vi "1473R Acquisition Template (Host).vi"() -> ()   [LabVIEW 2015]
uses:
  <vilib>/rvi/interface/nirviOpenFPGA/nirviOpenFPGA.xnode
  <vilib>/rvi/interface/nirviMethod/nirviMethod.xnode
  <vilib>/rvi/interface/nirviReadWriteControl/nirviReadWriteControl.xnode
  <vilib>/rvi/interface/nirviCloseFPGA/nirviCloseFPGA.xnode
  <vilib>/rvi/interface/Simulation/niFpgaSimulationCallBeginRW.vi
  <vilib>/rvi/errors/niLvFpgaAdjustHostInterfaceError.vi
  <vilib>/FPGAPlugInAG/Dynamic/niLvFpga_Run_Dynamic.vi
  <vilib>/FPGAPlugInAG/Dynamic/niLvFpga_Close_Dynamic.vi
  <vilib>/visionFPGA/NI_VDM_FPGA_Basics.lvlib
  <vilib>/visionFPGA/Basics/Configure Image Transfer from Target/IMAQ FPGA Configure Image Transfer from Target U8.vi
  <vilib>/FPGAPlugInAG/Dynamic/niLvFpga_Download_Dynamic.vi
  <vilib>/visionFPGA/Basics/Image Transfer from Target/IMAQ FPGA Image Transfer from Target U8.vi
  NiFpgaLv.dll
  <vilib>/Utility/error.llb/Error Cluster From Error Code.vi
  FPGA Bitfiles/ImageProcessingw_FPGATarget1_ImageProcessingw_ENrq3A+Q5NY.lvbitx
  Image Processing with Vision Assistant on 1473R (FPGA).vi
  <vilib>/FPGAPlugInAG/PCIe-1473R/niLvFpga_Open_PCIe-1473R.vi
  <vilib>/rvi/interface/common/dynamic/niFpgaDynamicAddResources.vi
  <vilib>/userdefined/Silver/nirio_resource_slv.ctl
panel:
  in  "Image Size":cluster{"Height":u32, "Width":u32}
  out "Acq In Progress":bool
  in  "Line Scan":bool
  in  "Frames To Acquire":u32=1 caption="Frames To Acquire\n(0 = infinite)"
  in  "Cancel":bool
  out "Acq'd Frame Width":u32
  in  "Stopped":bool
  in  "RIO Device":T1="RIO0"
  out "Acquisition Overflow":bool
  in  "Start Serial Server":bool=TRUE
  out "Frames Acq'd":u32
  out "Acq'd Frame Height":u32
  out "Image":T2(plugin-control)
  in  "Acquire":bool
  in  "Stop":bool
  out "Initialized":bool
  # "Overview: Demonstrates how to acquire an image from a Camera Link camera using the 1473R, process the image on the FPGA using the Vision Assistant Express VI, and transfer the processed image to the host.  Additionally, the example demonstrates the serial server, which allows third-party camera configuration utilities to communicate with the camera using the Camera Link serial interface while this VI is running.\nRequirements:\n- LabVIEW FPGA\n- Vision Acquisition Software\n- Vision Development Module\nInstructions:\n1. Select the RIO Device corresponding to the 1473R.\n2. Set the image size controls to the expected size of the image from the camera.\n3. Run the VI."
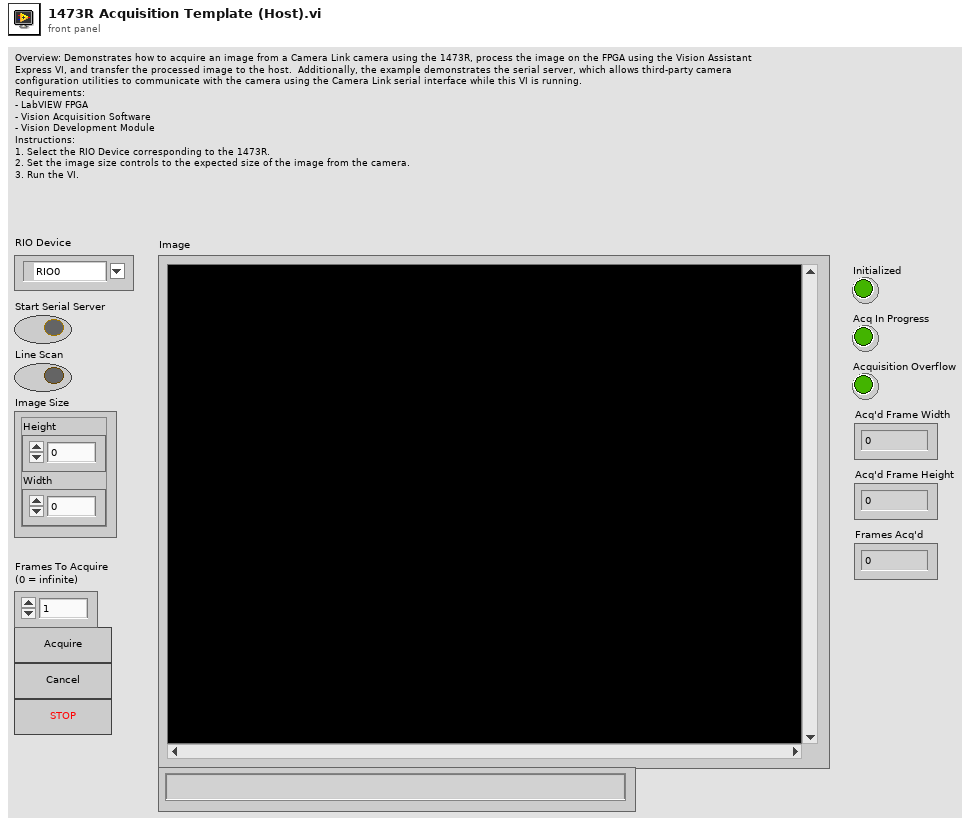
[diagram p1: front panel]
types:
  T1 = typedef "nirio_resource_slv.ctl" = tag
  T2 = typedef "IMAQ Image.ctl" = refnum<image>
  T3 = enum8{"Standard", "Basler 10-tap", "Vosskühler 10-tap"}
  T4 = typedef "Image Type" = u32
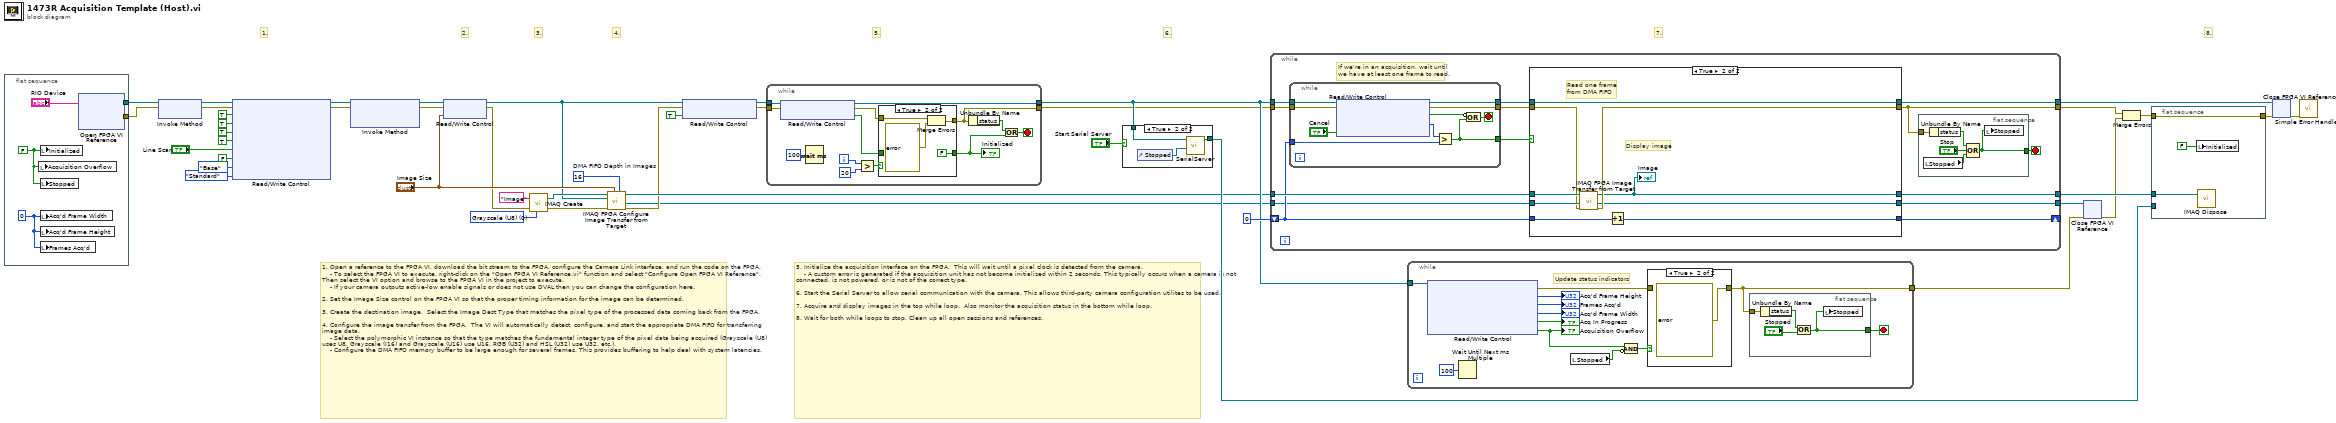
[diagram p0: block diagram]
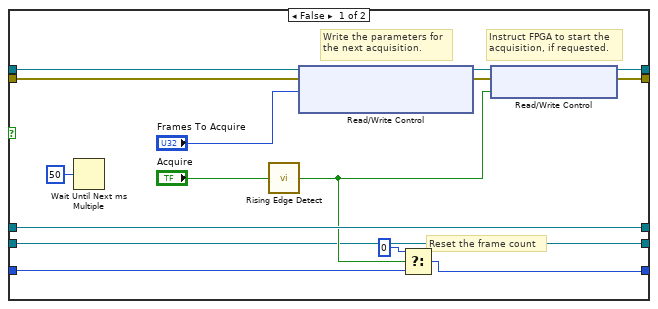
[diagram p4: hidden frame]
diagram:
  w12 = u32 16  # DMA FIFO Depth in Images
  w40 = T4 0 items=["Grayscale (U8)", "Grayscale (I16)", "Grayscale (SGL)", "Complex (CSG)", "RGB (U32)", "HSL (U32)", "RGB (U64)", "Grayscale (U16)"] ("Image Type")
  # "8."
  # "7."
  # "6."
  # "5."
  # "4."
  # "3."
  # "2."
  # "1."
  # "5. Initialize the acquisition interface on the FPGA.  This will wait until a pixel clock is detected from the camera.\n    - A custom error is generated if the acquisition unit has not become initialized within 2 seconds. This typically occurs when a camera is not connected, is not powered, or is not of the correct type.\n\n6. Start the Serial Server to allow serial communication with the camera. This allows third-party camera configuration utilites to be used.\n\n7. Acquire and display images in the top while loop.  Also monitor the acquisition status in the bottom while loop.\n\n8. Wait for both while loops to stop. Clean up all open sessions and references."
  # "1. Open a reference to the FPGA VI, download the bit stream to the FPGA, configure the Camera Link interface, and run the code on the FPGA.\n    - To select the FPGA VI to execute, right-click on the \"Open FPGA VI Reference.vi\" function and select \"Configure Open FPGA VI Reference\".  Then select the VI option and browse to the FPGA VI in the project to execute.\n    - If your camera outputs active-low enable signals or does not use DVAL then you can change the configuration here. \n\n2. Set the Image Size control on the FPGA VI so that the proper timing information for the image can be determined.\n\n3. Create the destination image.  Select the Image Dest Type that matches the pixel type of the processed data coming back from the FPGA.\n\n4. Configure the image transfer from the FPGA.  The VI will automatically detect, configure, and start the appropriate DMA FIFO for transferring image data.  \n    - Select the polymorphic VI instance so that the type matches the fundamental integer type of the pixel data being acquired (Grayscale (U8) uses U8, Grayscale (I16) and Grayscale (U16) use U16, RGB (U32) and HSL (U32) use U32, etc.).\n    - Configure the DMA FIFO memory buffer to be large enough for several frames. This provides buffering to help deal with system latencies."
  n1 = flat-sequence {
    tunnel: [w46] -> w36
    tunnel: [w45] -> w44
    frame #0 {
      w49 = u32 0 ("Num Lines Acq'd")
      w48 = FALSE ("stop")
      n2 = local write "Acquisition Overflow"(w48) -> ()
      n3 = local write "Initialized"(w48) -> ()
      n4 = local write "Stopped"(w48) -> ()
      n5 = local write "Acq'd Frame Width"(w49) -> ()
      n6 = local write "Acq'd Frame Height"(w49) -> ()
      n7 = local write "Frames Acq'd"(w49) -> ()
      n8 = xnode "Open FPGA VI Reference"("resource name"="RIO Device") -> ("FPGA VI Reference Out"=w46:refnum<k20>, "error out"=w45:errorcluster)  [unwired: 1 in]
    }
  }
  n9 = xnode "Invoke Method"("FPGA VI Reference In"=w36, "error in"=w44) -> ("FPGA VI Reference Out"=w29:refnum<k20>, "error out"=w32:errorcluster)
  n10 = xnode "Read/Write Control"("FPGA VI Reference In"=w29, "error in"=w32, "CL Config.FVAL Active High"=TRUE ("IO Module Config.CL FVAL Active High"), "CL Config.LVAL Active High"=TRUE ("IO Module Config.CL LVAL Active High"), "CL Config.DVAL Active High"=TRUE ("IO Module Config.CL DVAL Active High"), "CL Config.Spare Active High"=TRUE ("IO Module Config.CL Spare Active High"), "CL Config.Line Scan"="Line Scan", "Acq Control.Ignore DVAL"=FALSE ("CL Config.Line Scan"), "CL Config.Configuration"=enum8{"Base", "Medium", "Full"}."Base", "CL Config.Signal Mapping"=T3."Standard") -> ("FPGA VI Reference Out"=w33:refnum<k20>, "error out"=w31:errorcluster)
  n11 = xnode "Invoke Method"("FPGA VI Reference In"=w33, "error in"=w31) -> ("FPGA VI Reference Out"=w15:refnum<k20>, "error out"=w14:errorcluster)  [unwired: 1 in]
  n12 = xnode "Read/Write Control"("FPGA VI Reference In"=w15, "error in"=w14, "Image Size"="Image Size") -> ("FPGA VI Reference Out"=w1:refnum<k20>, "error out"=w8:errorcluster)
  n13 = call "IMAQ Create"("Image Name"="Image", "Image Type"=w40, "error in (no error)"=w8) -> ("New Image"=w11:T2, "error out"=w9:errorcluster)  [unwired: 2 in]
  n14 = call-poly <vilib>:"IMAQ FPGA Configure Image Transfer from Target.vi"("DMA FIFO Depth in Images"=w12, "Image Size"="Image Size", "error in (no error)"=w9, "FPGA VI Reference In"=w1, "Image"=w11) -> ("error out"=w7:errorcluster, "DMA FIFO Reference Out"=w5:refnum<k20>, "Image Out"=w10:T2)  [unwired: 4 in]
  n15 = xnode "Read/Write Control"("FPGA VI Reference In"=w1, "error in"=w7, "Acq Control.Initialize"=TRUE ("Arm Acquisition")) -> ("FPGA VI Reference Out"=w43:refnum<k20>, "error out"=w42:errorcluster)
  n16 = while {
    tunnel: w43 -> [w57]
    tunnel: w42 -> [w56]
    tunnel: [w55] -> w23
    tunnel: [w59] -> w6
    i -> [w51]
    stop <- w62 stop-if-true
    n17 = xnode "Read/Write Control"("FPGA VI Reference In"=w57, "error in"=w56) -> ("FPGA VI Reference Out"=w55:refnum<k20>, "error out"=w54:errorcluster, "Acq Status.Initialized"=w53:bool)
    n18 = Wait (ms)(milliseconds to wait=u32 100) -> ()  [unwired: 1 out]
    n19 = Greater?(x=w51, y=20) -> (0:w52:bool)
    n20 = case shown="True" w52 {
      tunnel: [w64 FALSE] -> w58
      tunnel: w53 -> [w64 _]
      tunnel: w54 -> [w63 w66]
      tunnel: [w63 w68] -> w59
      frame False {
      }
      frame True {
        n21 = Merge Errors(w66, errorcluster {"status"=TRUE, "code"=-8999, "source"="Acquisition Initialization: This error typically occurs when a camera is not properly connected, is not powered, or is not of the correct type."} ("error in")) -> (w68:errorcluster)
      }
    }
    "Initialized" <- w58
    n22 = Unbundle By Name(w59) -> ("status"=w61:bool)
    n23 = Or(x=w61, y=w58) -> (x .or. y?=w62:bool)
  }
  n24 = case shown="True" "Start Serial Server" {
    tunnel: [_ w69] -> w37
    tunnel: w23 -> [_ w70]
    frame False {
    }
    frame True {
      n25 = control-ref of="Stopped"() -> (w71:refnum<vi>)
      n26 = call "SerialServer.vi"("Stop Refnum"=w71, "FPGA VI Reference In"=w70) -> ("FPGA VI Reference Out"=w69:refnum<k20>)  [unwired: 5 in]
    }
  }
  n27 = while {
    tunnel: w23 -> [w80]
    tunnel: w6 -> [w79]
    tunnel: w10 -> [w85]
    tunnel: [w83] -> w34
    tunnel: [w84] -> w20
    tunnel: [w81] -> w38
    shift-right: [w72] -> _
    shift-left: u32 0 -> [w75]
    tunnel: w5 -> [w74]
    tunnel: [w73] -> w4
    stop <- w82 stop-if-true
    # "If we're in an acquisition, wait until\nwe have at least one frame to read."
    n28 = while {
      tunnel: w80 -> [w92]
      tunnel: w79 -> [w91]
      tunnel: [w89] -> w78
      tunnel: [w90] -> w77
      tunnel: w75 -> [w95]
      tunnel: [w93] -> w76
      stop <- w94 stop-if-true
      n29 = xnode "Read/Write Control"("FPGA VI Reference In"=w92, "error in"=w91, "Acq Control.Cancel Acq"="Cancel") -> ("FPGA VI Reference Out"=w90:refnum<k20>, "error out"=w89:errorcluster, "Acq Status.Acq In Progress"=w88:bool, "Acq Status.Frames Acq'd"=w87:u32)
      n30 = Greater?(x=w87, y=w95) -> (0:w93:bool)
      n31 = Compound Arithmetic op=OR(invert w88, w93) -> (w94:bool)
    }
    n32 = case shown="True" w76 {
      tunnel: w77 -> [w111 w122]
      tunnel: w78 -> [w110 w119]
      tunnel: w85 -> [w115 w121]
      tunnel: [w105 w118] -> w83
      tunnel: [w108 w122] -> w84
      tunnel: [w115 w116] -> w81
      tunnel: w75 -> [w112 w124]
      tunnel: [w114 w123] -> w72
      tunnel: w74 -> [w101 w120]
      tunnel: [w101 w117] -> w73
      frame False {
        # "Reset the frame count"
        # "Instruct FPGA to start the\nacquisition, if requested."
        # "Write the parameters for\nthe next acquisition."
        n33 = Wait Until Next ms Multiple(millisecond multiple=u32 50) -> ()  [unwired: 1 out]
        n34 = call "Rising Edge Detect.vi"("Input"="Acquire") -> ("Pulse"=w102:bool)  [unwired: 4 in]
        n35 = xnode "Read/Write Control"("FPGA VI Reference In"=w111, "error in"=w110, "Acq Control.Frames To Acq"="Frames To Acquire") -> ("FPGA VI Reference Out"=w107:refnum<k20>, "error out"=w106:errorcluster)  [unwired: 1 in]
        n36 = Select(t=u32 0, s=w102, f=w112) -> (s? t:f=w114:u32)
        n37 = xnode "Read/Write Control"("FPGA VI Reference In"=w107, "error in"=w106, "Acq Control.Acquire"=w102) -> ("FPGA VI Reference Out"=w108:refnum<k20>, "error out"=w105:errorcluster)
      }
      frame True {
        # "Display image"
        # "Read one frame\nfrom DMA FIFO"
        n38 = call-poly <vilib>:"IMAQ FPGA Image Transfer from Target.vi"("error in (no error)"=w119, "DMA FIFO Reference In"=w120, "Image"=w121) -> ("error out"=w118:errorcluster, "DMA FIFO Reference Out"=w117:refnum<k20>, "Image Out"=w116:T2)  [unwired: 6 in]
        "Image" <- w116
        n39 = Increment(x=w124) -> (x+1=w123:u32)
      }
    }
    n40 = flat-sequence {
      tunnel: w83 -> [w98]
      tunnel: [w97] -> w82
      frame #0 {
        n41 = local read "Stopped"() -> (w96:bool)
        n42 = Unbundle By Name(w98) -> ("status"=w99:bool)
        n43 = Compound Arithmetic op=OR(w99, "Stop", w96) -> (w97:bool)
        n44 = local write "Stopped"(w97) -> ()
      }
    }
  }
  n45 = while {
    tunnel: w23 -> [w133]
    tunnel: [w136] -> w3
    stop <- w135 stop-if-true
    # "Update status indicators"
    n46 = xnode "Read/Write Control"("FPGA VI Reference In"=w133) -> ("error out"=w132:errorcluster, "Acq Status.Lines Per Frame"=→"Acq'd Frame Height":u32, "Acq Status.Frames Acq'd"=→"Frames Acq'd":u32, "Acq Status.Clocks Per Line"=→"Acq'd Frame Width":u32, "Acq Status.Acq In Progress"=→"Acq In Progress":bool, "Acq Status.Acquisition Overflow"=w126:bool)  [unwired: 1 in, 1 out]
    "Acquisition Overflow" <- w126
    n47 = Wait Until Next ms Multiple(millisecond multiple=u32 100) -> ()  [unwired: 1 out]
    n48 = local read "Stopped"() -> (w127:bool)
    n49 = Compound Arithmetic op=AND(w126, invert w127) -> (w125:bool)
    n50 = case shown="True" w125 {
      tunnel: w132 -> [w141 _]
      tunnel: [w141 errorcluster {"status"=TRUE, "code"=-8999, "source"="Acquisition Overflow: The write operation to the Acquisition FIFO on the FPGA timed out. This can be caused by the DMA FIFO not being started or the DMA FIFO overflowing. Make sure that Start is being called on the DMA FIFO. Also make sure that the host application is reading from the DMA FIFO fast enough to prevent it from overflowing."} ("error out")] -> w136
      frame False {
      }
      frame True {
      }
    }
    n51 = flat-sequence {
      tunnel: w136 -> [w140]
      tunnel: [w138] -> w135
      frame #0 {
        n52 = Unbundle By Name(w140) -> ("status"=w139:bool)
        n53 = Or(x=w139, y="Stopped") -> (x .or. y?=w138:bool)
        n54 = local write "Stopped"(w138) -> ()
      }
    }
  }
  n55 = xnode "Close FPGA VI Reference"("FPGA VI Reference In"=w4, "error in"=w3) -> ("error out"=w2:errorcluster)
  n56 = Merge Errors(w34, w2) -> (w35:errorcluster)
  n57 = flat-sequence {
    tunnel: w35 -> [w144]
    tunnel: [w144] -> w18
    tunnel: w38 -> [w145]
    tunnel: w37 -> [_]
    frame #0 {
      n58 = local write "Initialized"(FALSE ("Module Enabled")) -> ()
      n59 = call "IMAQ Dispose"("Image"=w145) -> ()  [unwired: 5 in, 1 out]
    }
  }
  n60 = xnode "Close FPGA VI Reference"("FPGA VI Reference In"=w20, "error in"=w18) -> ("error out"=w19:errorcluster)
  n61 = call <vilib>:"Simple Error Handler.vi"("error in (no error)"=w19) -> ()  [unwired: 4 in, 5 out]
